vi "Query Current.vi"(8 "error in (no error)":errorcluster, 11 "E364x in":refnum<class "E364x.lvclass">) -> (0 "error out":errorcluster, 2 "Current":dbl, 3 "E364x out":refnum<class "E364x.lvclass">)   [LabVIEW 2020, in "E364x.lvclass"]
uses:
  E364x.lvclass
  C:/Sandbox/Git_Sandbox/WiSpry Test Framework source code (LV20)/WiSpry Test Framework/Instruments/Instrument.lvclass
  Instrument.lvclass/Instrument.ctl
  Instrument.lvclass
  <instrlib>/Agilent E364X Series/Agilent E364X Series.lvlib
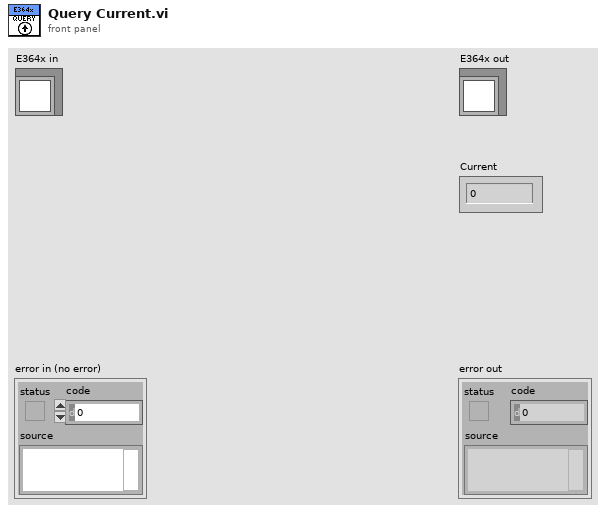
[diagram p1: front panel]
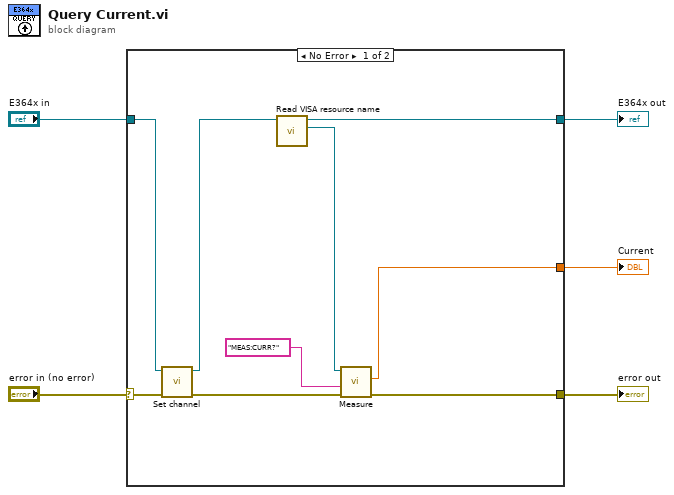
[diagram p0: block diagram]
diagram:
  n1 = case shown="No Error" "error in (no error)" {
    selector: "error in (no error)" -> [w9 w16]
    tunnel: [w11 w16] -> w4
    tunnel: "E364x in" -> [w7 w15]
    tunnel: [w12 w15] -> w2
    tunnel: [w10 _] -> w1
    frame No Error {
      n2 = call "Set channel.vi"("error in (no error)"=w9, "E364x in"=w7) -> ("error out"=w8:errorcluster, "E364x out"=w6:refnum<class "E364x.lvclass">)  [unwired: 7 in, 1 out]
      n3 = call "Read VISA resource name.vi"("Instrument in"=w6) -> ("VISA resource name"=w13:refnum<visa-resource-name>, "Instrument out"=w12:refnum<class "E364x.lvclass">)  [unwired: 9 in]
      n4 = call <instrlib>:"Measure.vi"("error in (no error)"=w8, "Measurement Type (Voltage)"="MEAS:CURR?", "VISA resource name"=w13) -> ("error out"=w11:errorcluster, "Measurement"=w10:dbl)  [unwired: 6 in, 1 out]
    }
    frame Error {
    }
  }
  "error out" <- w4
  "E364x out" <- w2
  "Current" <- w1
